vi "Teleop.vi"(10 "Match Info":T1={"Autonomous Elapsed Seconds"=0.0, "TeleOp Elapsed Seconds"=0.0, "Disabled Elapsed Seconds"=0.0, "Visited Autonomous"=FALSE, "Visited TeleOp"=FALSE, "Visited Disabled"=FALSE, "Autonomous Settings"={"Autonomous Style"=enum."Independent", "VI Refnum"=refnum}}, 11 "Call Context":T2) -> ()   [LabVIEW 2017]
doc: "This VI is called for each TeleOp packet received from the DS where the robot is not disabled. It is often used to read from the joysticks and update I/O or to update setpoints for timed control loops. It should complete and return within 20 milliseconds or it may miss DS packets."
uses:
  <vilib>/Rock Robotics/WPI/DriverStation/WPI_DriverStationDerivedRobotMode.ctl
  <vilib>/Rock Robotics/WPI/DriverStation/WPI_DriverStationMatch Info.ctl
  <vilib>/Rock Robotics/Network Tables/NT Read Boolean.vi
  <vilib>/Rock Robotics/Network Tables/NT Read Number.vi
  <vilib>/Rock Robotics/WPI/Utilities/WPI_GetSetVariantRefNum.vi
  <vilib>/Rock Robotics/Network Tables/NT Write Boolean Array.vi
  <vilib>/Rock Robotics/Network Tables/NT Write Numeric Array.vi
  Robot Global Data.vi
panel:
  out "Sample Slider 0":dbl(slide) scale=0.0..5.0
  out "Sample Boolean 1":bool
  out "Sample Boolean 0":bool
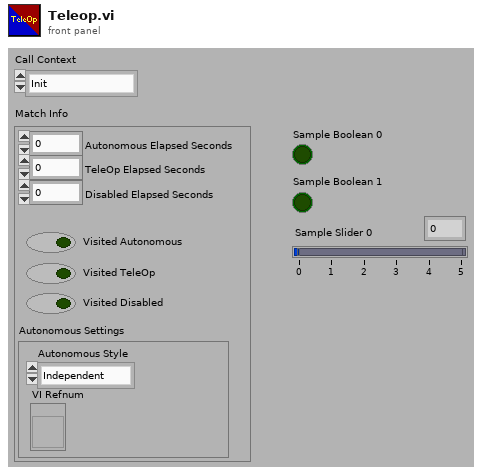
[diagram p1: front panel]
types:
  T1 = typedef "WPI_DriverStationMatch Info.ctl" = cluster{"Autonomous Elapsed Seconds":dbl, "TeleOp Elapsed Seconds":dbl, "Disabled Elapsed Seconds":dbl, "Visited Autonomous":bool, "Visited TeleOp":bool, "Visited Disabled":bool, "Autonomous Settings":cluster{"Autonomous Style":enum16{"Iterative", "Independent"}, "VI Refnum":refnum<vi>}}
  T2 = typedef "WPI_DriverStationDerivedRobotMode.ctl" = enum16{"Init", "Execute", "Stop"}
  T3 = typedef "WPI_JoystickDevRef.ctl" = cluster{"Device":T4}
  T4 = typedef "WPI_JoystickDeviceEnum.ctl" = enum16{"USB 0", "USB 1", "USB 2", "USB 3", "USB 4", "USB 5"}
  T5 = typedef "Control 1.ctl" = enum16{"SingleJoystick", "DoubleJoystick", "GameController"}
  T6 = cluster{"Buttons[0]":bool, "Buttons[1]":bool, "Buttons[2]":bool, "Buttons[3]":bool, "Buttons[4]":bool, "Buttons[5]":bool, "Buttons[6]":bool, "Buttons[7]":bool, "Buttons[8]":bool}
  T7 = cluster{"Axes[0]":dbl, "Axes[1]":dbl, "Axes[2]":dbl, "Axes[3]":dbl, "Axes[4]":dbl, "Axes[5]":dbl, "Axes[6]":dbl, "Axes[7]":dbl, "Axes[8]":dbl}
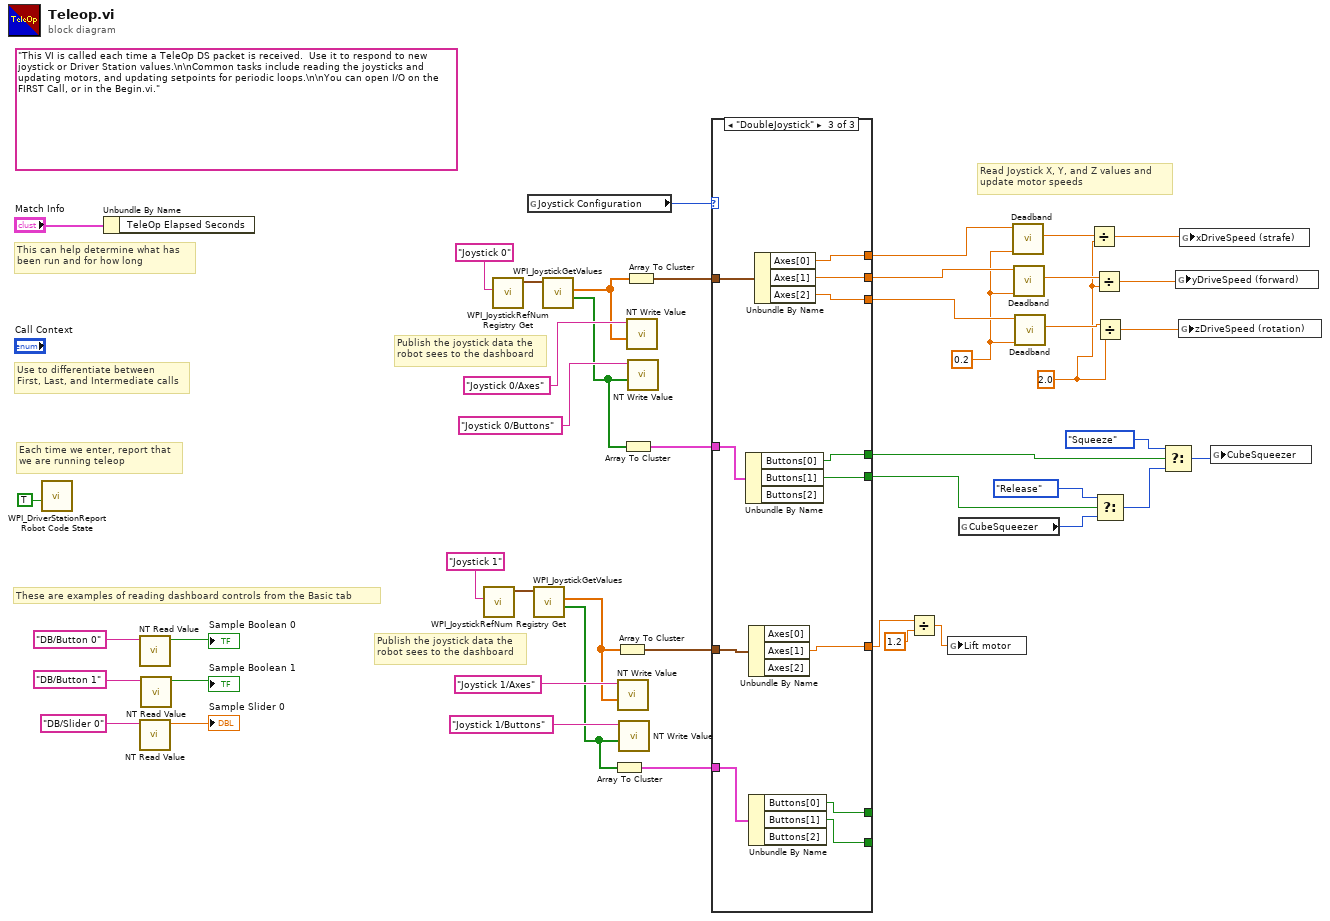
[diagram p0: block diagram]
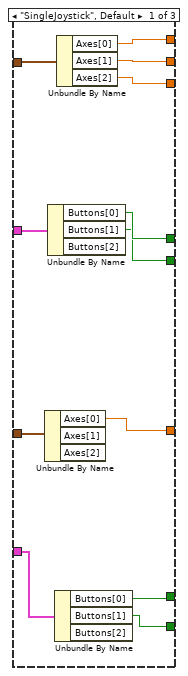
[diagram p2: hidden frame]
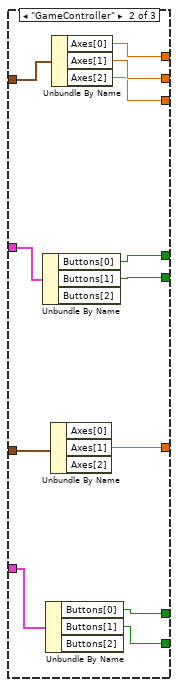
[diagram p3: hidden frame]
diagram:
  w7 = 2.0
  w25 = 0.2 ("guardband value")
  (unwired) "This VI is called each time a TeleOp DS packet is received.  Use it to respond to new joystick or Driver Station values.\n\nCommon tasks include reading the joysticks and updating motors, and updating setpoints for periodic loops.\n\nYou can open I/O on the FIRST Call, or in the Begin.vi."
  # "Publish the joystick data the\nrobot sees to the dashboard"
  # "Publish the joystick data the\nrobot sees to the dashboard"
  # "Read Joystick X, Y, and Z values and \nupdate motor speeds"
  # "These are examples of reading dashboard controls from the Basic tab"
  # "Each time we enter, report that\nwe are running teleop"
  # "Use to differentiate between\nFirst, Last, and Intermediate calls"
  # "This can help determine what has\nbeen run and for how long"
  n1 = call <vilib>:"WPI_DriverStationReport Robot Code State.vi"("TeleOp"=TRUE ("Autonomous")) -> ()  [unwired: 10 in, 1 out]
  n2 = Unbundle By Name("Match Info") -> ()  [unwired: 1 out]
  n3 = call-poly <vilib>:"NT Read Value.vi"("Name"="DB/Button 0" ("refnum name")) -> ("Boolean"=→"Sample Boolean 0":bool)  [unwired: 9 in, 1 out]
  n4 = call-poly <vilib>:"NT Read Value.vi"("Name"="DB/Slider 0" ("refnum name")) -> ("Numeric"=→"Sample Slider 0":dbl)  [unwired: 9 in, 1 out]
  n5 = call-poly <vilib>:"NT Read Value.vi"("Name"="DB/Button 1" ("refnum name")) -> ("Boolean"=→"Sample Boolean 1":bool)  [unwired: 9 in, 1 out]
  n6 = call <vilib>:"WPI_JoystickRefNum Registry Get.vi"("refnum name"="Joystick 1") -> ("JoystickDevRef"=w18:T3)  [unwired: 1 in, 9 out]
  n7 = call <vilib>:"WPI_JoystickRefNum Registry Get.vi"("refnum name"="Joystick 0") -> ("JoystickDevRef"=w37:T3)  [unwired: 1 in, 9 out]
  n8 = global read "Robot Global Data.vi" "Joystick Configuration"() -> (w11:T5)
  n9 = call <vilib>:"WPI_JoystickGetValues.vi"("JoystickDevRef"=w18) -> ("Buttons"=w13:bool[], "Axes"=w15:dbl[])  [unwired: 6 in, 3 out]
  n10 = call <vilib>:"WPI_JoystickGetValues.vi"("JoystickDevRef"=w37) -> ("Buttons"=w32:bool[], "Axes"=w34:dbl[])  [unwired: 6 in, 3 out]
  n11 = Array To Cluster(array=w13) -> (cluster=w12:T6)
  n12 = Array To Cluster(array=w15) -> (cluster=w14:T7)
  n13 = call-poly <vilib>:"NT Write Value.vi"("Numeric Array"=w15, "Name"="Joystick 1/Axes") -> ()  [unwired: 9 in, 1 out]
  n14 = call-poly <vilib>:"NT Write Value.vi"("Boolean Array"=w13, "Name"="Joystick 1/Buttons") -> ()  [unwired: 9 in, 1 out]
  n15 = Array To Cluster(array=w32) -> (cluster=w31:T6)
  n16 = Array To Cluster(array=w34) -> (cluster=w33:T7)
  n17 = call-poly <vilib>:"NT Write Value.vi"("Numeric Array"=w34, "Name"="Joystick 0/Axes") -> ()  [unwired: 9 in, 1 out]
  n18 = call-poly <vilib>:"NT Write Value.vi"("Boolean Array"=w32, "Name"="Joystick 0/Buttons") -> ()  [unwired: 9 in, 1 out]
  n19 = case shown="\"DoubleJoystick\"" w11 {
    tunnel: w33 -> [w58 w70 w82]
    tunnel: w31 -> [w57 w69 w81]
    tunnel: [w56 w68 w80] -> w30
    tunnel: [w55 w67 w79] -> w29
    tunnel: [w54 w66 w78] -> w28
    tunnel: [w53 w65 w77] -> w27
    tunnel: [w52 w64 w76] -> w26
    tunnel: w14 -> [w48 w60 w75]
    tunnel: w12 -> [w51 w63 w74]
    tunnel: [w50 w62 w73] -> _
    tunnel: [w49 w61 w72] -> _
    tunnel: [w47 w59 w71] -> w3
    frame "SingleJoystick", Default {
      n20 = Unbundle By Name(w48) -> ("Axes[0]"=w47:dbl)  [unwired: 2 out]
      n21 = Unbundle By Name(w57) -> ("Buttons[0]"=w53:bool, "Buttons[1]"=w52:bool)  [unwired: 1 out]
      n22 = Unbundle By Name(w51) -> ("Buttons[0]"=w50:bool, "Buttons[1]"=w49:bool)  [unwired: 1 out]
      n23 = Unbundle By Name(w58) -> ("Axes[0]"=w56:dbl, "Axes[1]"=w55:dbl, "Axes[2]"=w54:dbl)
    }
    frame "GameController" {
      n24 = Unbundle By Name(w69) -> ("Buttons[0]"=w65:bool, "Buttons[1]"=w64:bool)  [unwired: 1 out]
      n25 = Unbundle By Name(w63) -> ("Buttons[0]"=w62:bool, "Buttons[1]"=w61:bool)  [unwired: 1 out]
      n26 = Unbundle By Name(w60) -> ("Axes[1]"=w59:dbl)  [unwired: 2 out]
      n27 = Unbundle By Name(w70) -> ("Axes[0]"=w68:dbl, "Axes[1]"=w67:dbl, "Axes[2]"=w66:dbl)
    }
    frame "DoubleJoystick" {
      n28 = Unbundle By Name(w81) -> ("Buttons[0]"=w77:bool, "Buttons[1]"=w76:bool)  [unwired: 1 out]
      n29 = Unbundle By Name(w75) -> ("Axes[1]"=w71:dbl)  [unwired: 2 out]
      n30 = Unbundle By Name(w74) -> ("Buttons[0]"=w73:bool, "Buttons[1]"=w72:bool)  [unwired: 1 out]
      n31 = Unbundle By Name(w82) -> ("Axes[0]"=w80:dbl, "Axes[1]"=w79:dbl, "Axes[2]"=w78:dbl)
    }
  }
  n32 = Divide(x=w3, y=1.2) -> (x/y=w1:dbl)
  n33 = global write "Robot Global Data.vi" "Lift motor"(w1) -> ()
  n34 = global read "Robot Global Data.vi" "CubeSqueezer"() -> (w24:enum16{"Squeeze", "Release"})
  n35 = call "Deadband.vi"("+- Bounds"=w25, "Raw Value"=w30) -> ("Filtered Value"=w10:dbl)  [unwired: 9 in]
  n36 = call "Deadband.vi"("+- Bounds"=w25, "Raw Value"=w29) -> ("Filtered Value"=w9:dbl)  [unwired: 9 in]
  n37 = call "Deadband.vi"("+- Bounds"=w25, "Raw Value"=w28) -> ("Filtered Value"=w8:dbl)  [unwired: 9 in]
  n38 = Divide(x=w10, y=w7) -> (x/y=w4:dbl)
  n39 = Divide(x=w9, y=w7) -> (x/y=w5:dbl)
  n40 = Divide(x=w8, y=w7) -> (x/y=w6:dbl)
  n41 = Select(t=enum16{"Squeeze", "Release"}."Release" ("CubeSqueezer"), s=w26, f=w24) -> (s? t:f=w20:enum16{"Squeeze", "Release"})
  n42 = Select(t=enum16{"Squeeze", "Release"}."Squeeze" ("CubeSqueezer"), s=w27, f=w20) -> (s? t:f=w21:enum16{"Squeeze", "Release"})
  n43 = global write "Robot Global Data.vi" "yDriveSpeed (forward)"(w5) -> ()
  n44 = global write "Robot Global Data.vi" "zDriveSpeed (rotation)"(w6) -> ()
  n45 = global write "Robot Global Data.vi" "xDriveSpeed (strafe)"(w4) -> ()
  n46 = global write "Robot Global Data.vi" "CubeSqueezer"(w21) -> ()
